vi "Bar Code Reader_v6.vi"() -> ()   [LabVIEW 2016]
uses:
  <vilib>/NXT/Block Support/NXT_OutputPort.ctl
  <vilib>/NXT/Block Support/NXT_InputPort.ctl
  <vilib>/NXT/Dual Mode Library/Sensors/EV3_Color_Color.vi
  <vilib>/NXT/NXTIO Xnodes/NXTIONodeSubVIs/NXTMoveMotors.vi
  <vilib>/NXT/NXTIO Xnodes/NXTIONodeSubVIs/NXTMotorRunDistance.vi
  <vilib>/NXT/Dual Mode Library/Waits/Wait_Num.vi
  <vilib>/NXT/Subs/LVHSConnector.ctl
  <vilib>/NXT/NXTIO Xnodes/AddressXNode/NXTIOAddress.xnode
  <vilib>/NXT/NXTIO Xnodes/NXTIOXNode/NXTIO.xnode
  <vilib>/NXT/LegoClasses/BrickReference/BrickReference.lvclass
panel:
  out "Error Message":string
  out "Total Marbles":dbl
  out "Small/HDPE 4":dbl
  out "Large/Steel 4":dbl
  out "Material 4":string
  out "Small/HDPE 3":dbl
  out "Large/Steel 3":dbl
  out "Material 3":string
  out "Small/HDPE 2":dbl
  out "Large/Steel 2":dbl
  out "Material 2":string
  out "Small/HDPE 1":dbl
  out "Large/Steel 1":dbl
  out "String 3":string
  out "String 2":string
  out "Material 1":string
  out "String":string
  out "Numeric":dbl
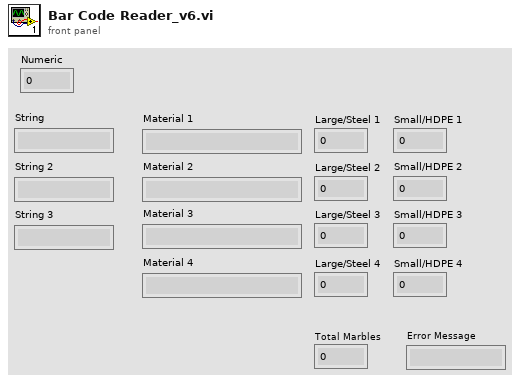
[diagram p1: front panel]
types:
  T1 = typedef "NXT_OutputPort.ctl" = u8
  T2 = typedef "ColorSensorColors.ctl" = enum16{"No Color", "Black", "Blue", "Green", "Yellow", "Red", "White", "Brown"}
  T3 = typedef "LVHSConnector.ctl" = refnum<class "BrickReference.lvclass">
  T4 = typedef "NXT_InputPort.ctl" = u32
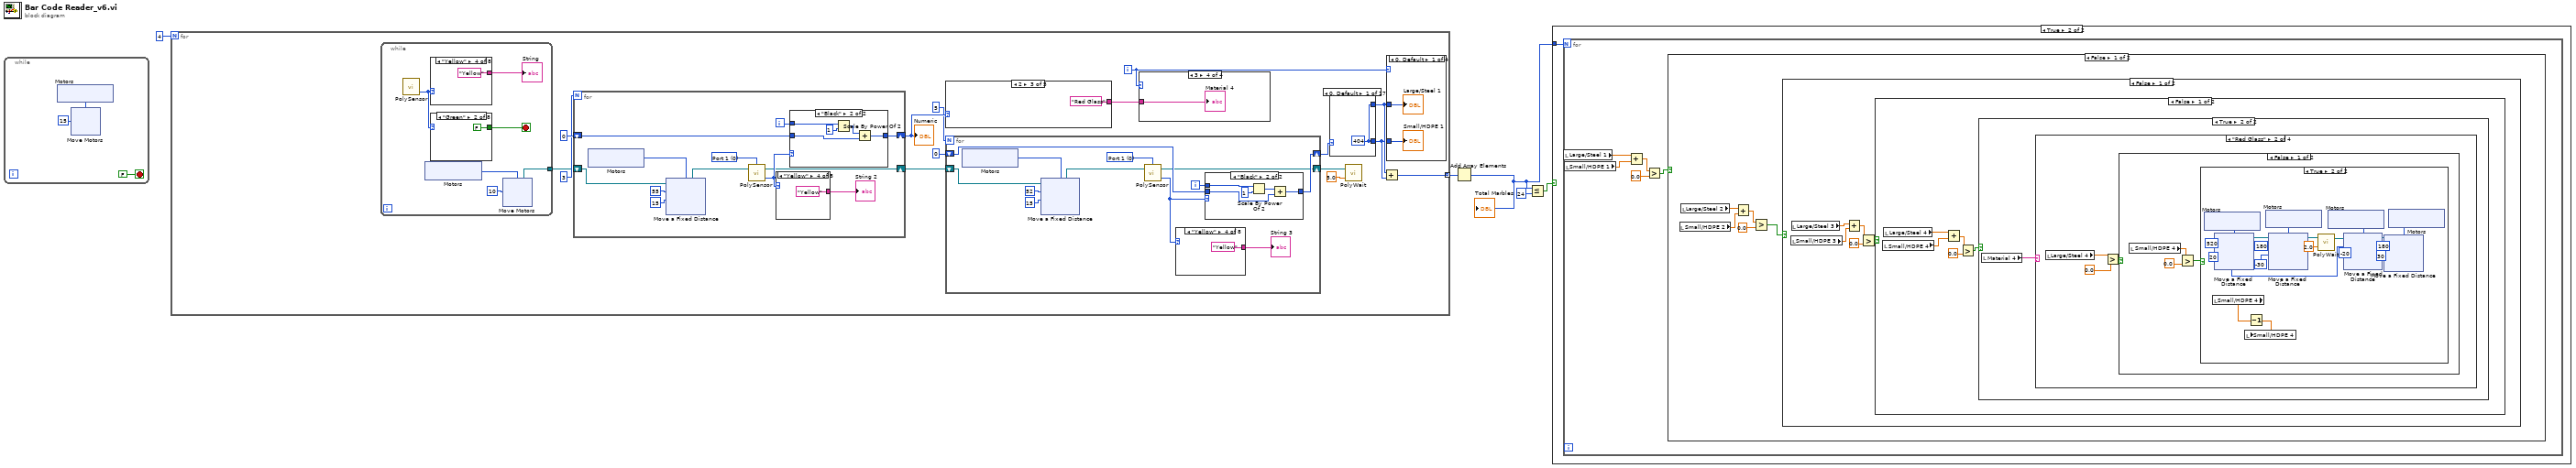
[diagram p0: block diagram]
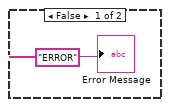
[diagram p2: hidden frame]
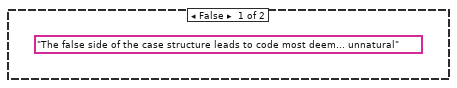
[diagram p3: hidden frame]
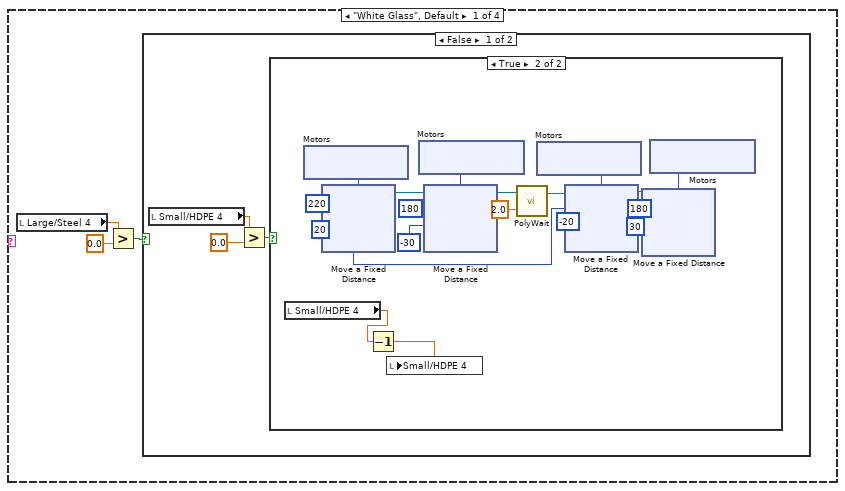
[diagram p4: hidden frame]
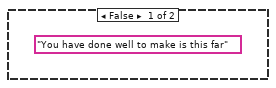
[diagram p5: hidden frame]
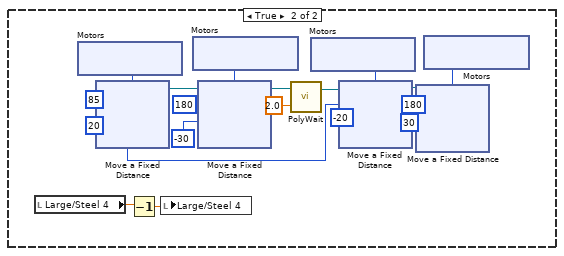
[diagram p6: hidden frame]
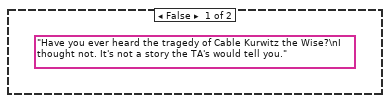
[diagram p7: hidden frame]
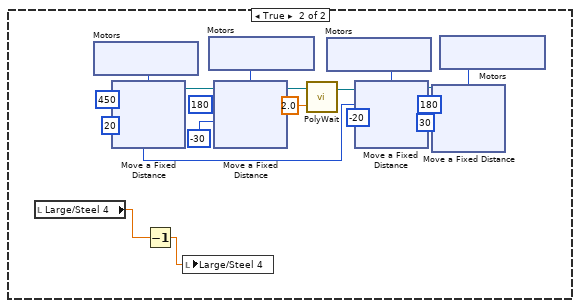
[diagram p8: hidden frame]
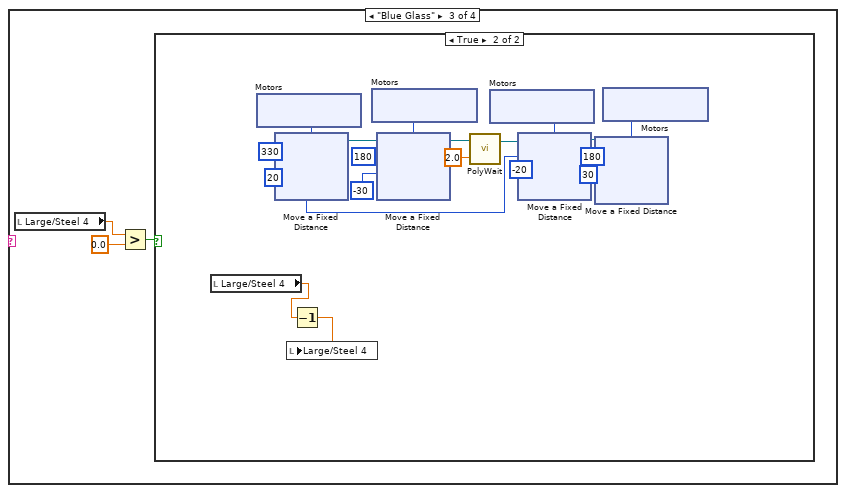
[diagram p9: hidden frame]
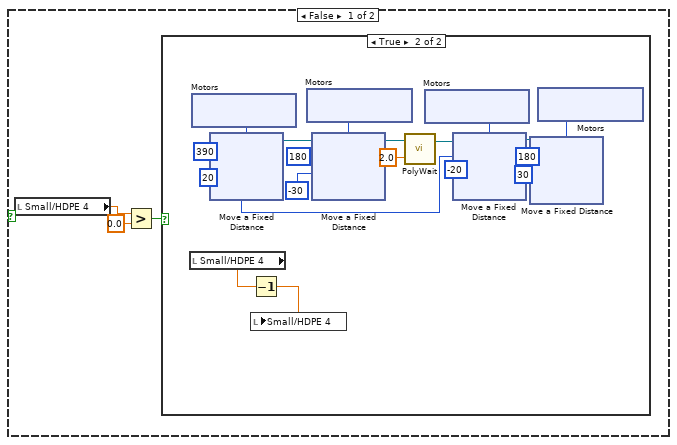
[diagram p10: hidden frame]
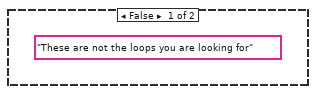
[diagram p11: hidden frame]
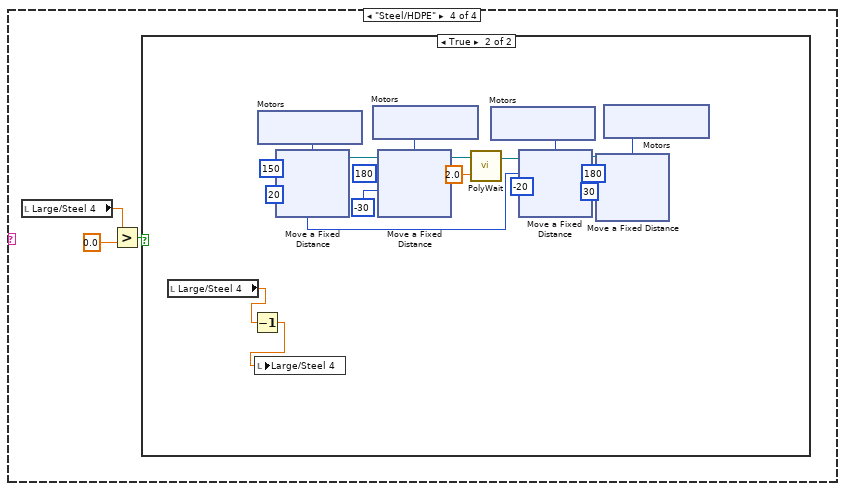
[diagram p12: hidden frame]
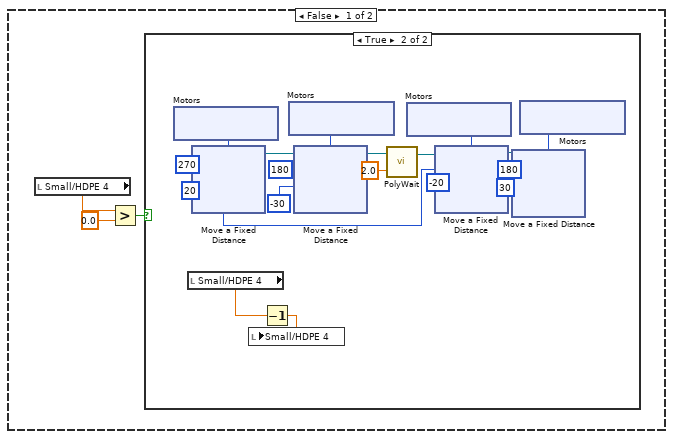
[diagram p13: hidden frame]
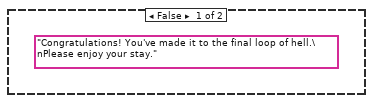
[diagram p14: hidden frame]
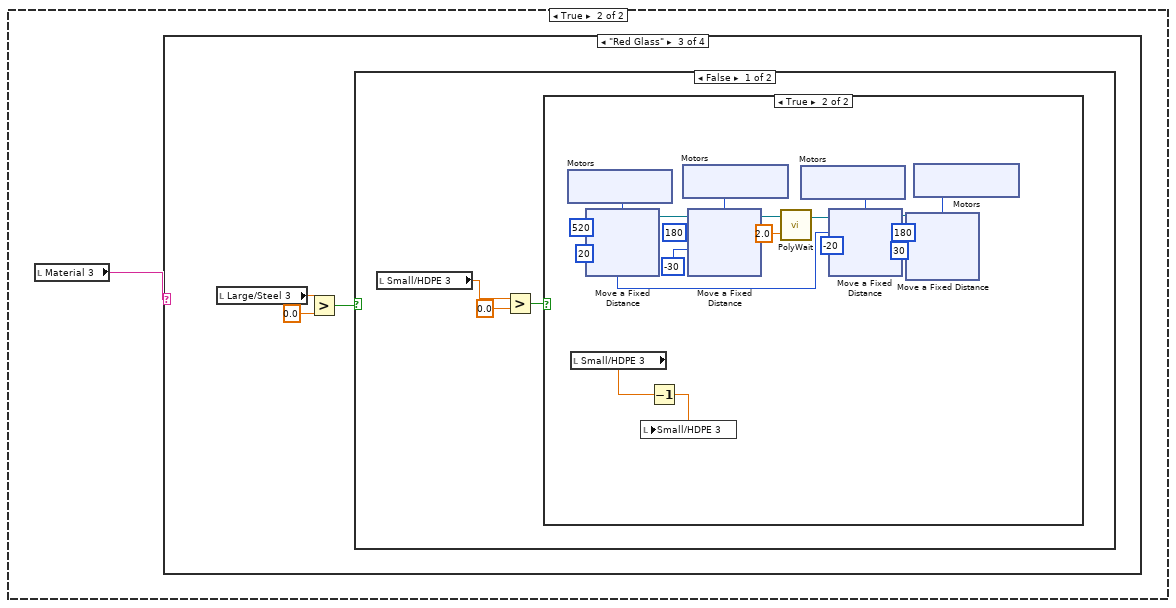
[diagram p15: hidden frame]
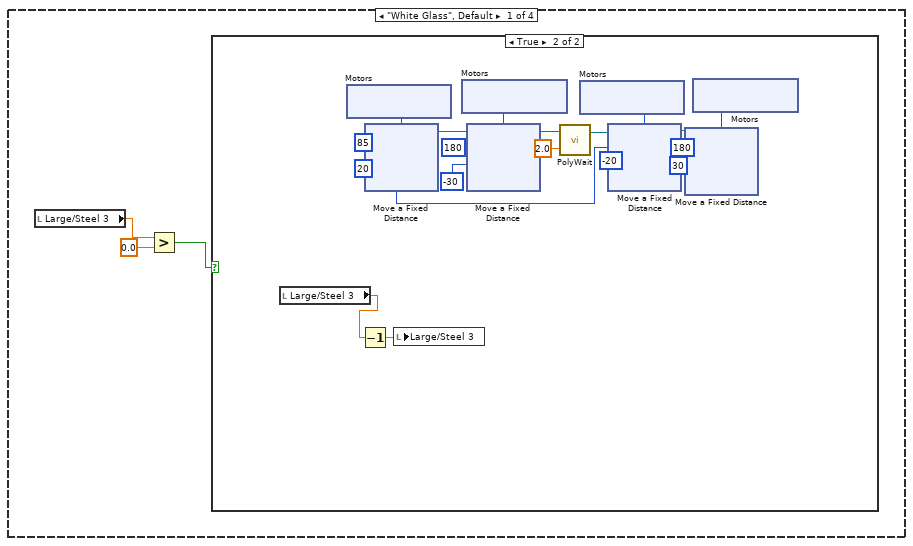
[diagram p16: hidden frame]
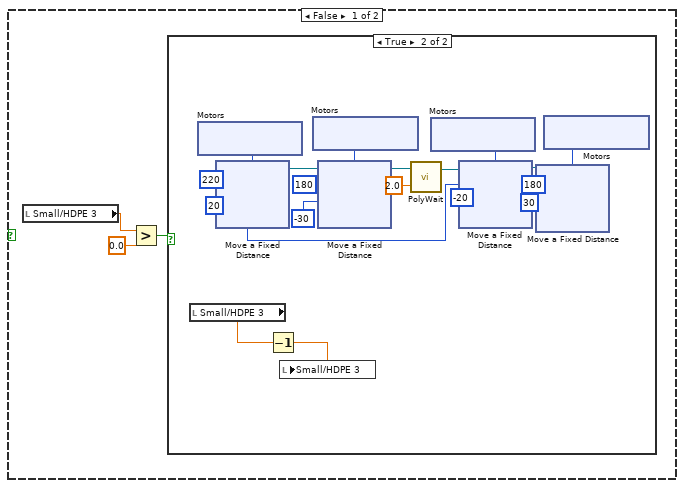
[diagram p17: hidden frame]
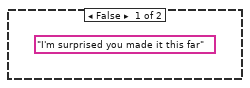
[diagram p18: hidden frame]
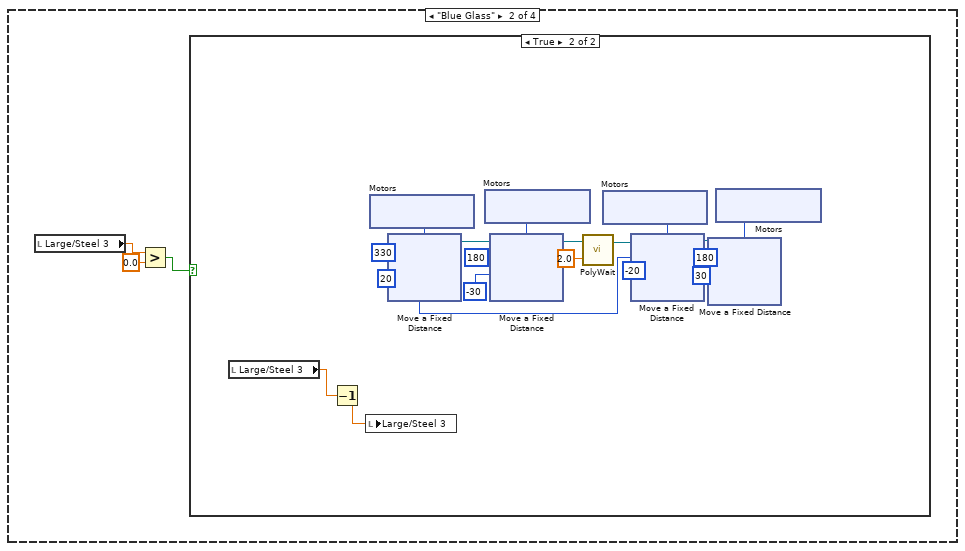
[diagram p19: hidden frame]
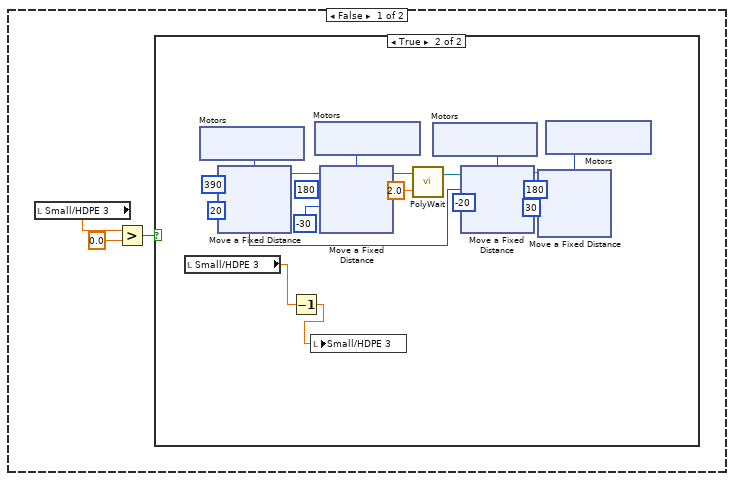
[diagram p20: hidden frame]
diagram:
  n1 = while {
    stop <- FALSE stop-if-true
    n2 = xnode "Motors"() -> ("Motor"=w6:T1)
    n3 = xnode "Move Motors"("Power/Speed 1"=i8 15, "Motors"=w6) -> ()  [unwired: 1 in, 1 out]
  }
  n4 = for {
    N: 4 -> [_]
    tunnel: [w17] -> w4 mode=indexing
    i -> [w22]
    n5 = while {
      tunnel: [w120] -> w29
      stop <- w124 stop-if-true
      n6 = call-poly <vilib>:"PolySensor.vi"() -> ("Detected Color"=w122:T2)  [unwired: 3 in, 1 out]
      n7 = xnode "Motors"() -> ("Motor"=w119:T1)
      n8 = case shown="\"Yellow\"" w122 {
        tunnel: ["No Color" "Blue" "Green" "Yellow" "Red" "White" "Brown" "Black"] -> w123
        frame "No Color", Default {
        }
        frame "Blue" {
        }
        frame "Green" {
        }
        frame "Yellow" {
        }
        frame "Red" {
        }
        frame "White" {
        }
        frame "Brown" {
        }
        frame "Black" {
        }
      }
      "String" <- w123
      n9 = case shown="\"Green\"" w122 {
        tunnel: [FALSE FALSE FALSE FALSE FALSE FALSE FALSE TRUE] -> w124
        frame "No Color", Default {
        }
        frame "Green" {
        }
        frame "Yellow" {
        }
        frame "Red" {
        }
        frame "White" {
        }
        frame "Brown" {
        }
        frame "Blue" {
        }
        frame "Black" {
        }
      }
      n10 = xnode "Move Motors"("Power/Speed 1"=i8 10, "Motors"=w119) -> ("NXT/EV3"=w120:T3)  [unwired: 1 in]
    }
    n11 = for {
      N: 3 -> [_]
      shift-right: [w160] -> w28
      shift-left: 0 -> [w159]
      shift-right: [w155] -> w24
      shift-left: w29 -> [w152]
      i -> [w156]
      w149 = T4 0 items=["Port 1", "Port 2", "Port 3", "Port 4"] ("Port (Port 1)")
      n12 = xnode "Motors"() -> ("Motor"=w150:T1)
      n13 = xnode "Move a Fixed Distance"("Speed 1"=i8 15, "Distance 1"=55, "Motors"=w150, "NXT/EV3"=w152) -> ("NXT/EV3"=w151:T3)
      n14 = call-poly <vilib>:"PolySensor.vi"("NXT/EV3"=w151, "Port (Port 1)"=w149) -> ("Detected Color"=w157:T2, "NXT/EV3"=w155:T3)  [unwired: 1 in]
      n15 = case shown="\"Yellow\"" w157 {
        tunnel: ["No Color" "Blue" "Green" "Yellow" "Red" "White" "Brown" "Black"] -> w158
        frame "No Color", Default {
        }
        frame "Blue" {
        }
        frame "Green" {
        }
        frame "Yellow" {
        }
        frame "Red" {
        }
        frame "White" {
        }
        frame "Brown" {
        }
        frame "Black" {
        }
      }
      "String 2" <- w158
      n16 = case shown="\"Black\"" w157 {
        tunnel: w156 -> [_ w184]
        tunnel: [w180 w182] -> w160
        tunnel: w159 -> [w180 w181]
        frame "White", Default {
        }
        frame "Black" {
          n17 = Scale By Power Of 2(n=w184, x=1) -> (x*2^n=w183:i32)
          n18 = Add(x=w183, y=w181) -> (x+y=w182:i32)
        }
      }
    }
    "Numeric" <- w28
    n19 = case shown="2" w28 {
      tunnel: ["Something has gone wrong" "White Glass" "Red Glass" "Blue Glass" "Steel/HDPE"] -> w27
      frame 0, Default {
      }
      frame 1 {
      }
      frame 2 {
      }
      frame 3 {
      }
      frame 4 {
      }
    }
    n20 = for {
      N: 5 -> [_]
      shift-right: [w88] -> w23
      shift-left: 0 -> [w87]
      shift-right: [w83] -> w21
      shift-left: w24 -> [w80]
      i -> [w84]
      w77 = T4 0 items=["Port 1", "Port 2", "Port 3", "Port 4"] ("Port (Port 1)")
      n21 = xnode "Motors"() -> ("Motor"=w78:T1)
      n22 = xnode "Move a Fixed Distance"("Speed 1"=i8 15, "Distance 1"=52, "Motors"=w78, "NXT/EV3"=w80) -> ("NXT/EV3"=w79:T3)
      n23 = call-poly <vilib>:"PolySensor.vi"("NXT/EV3"=w79, "Port (Port 1)"=w77) -> ("Detected Color"=w85:T2, "NXT/EV3"=w83:T3)  [unwired: 1 in]
      n24 = case shown="\"Yellow\"" w85 {
        tunnel: ["No Color" "Blue" "Green" "Yellow" "Red" "White" "Brown" "Black"] -> w86
        frame "No Color", Default {
        }
        frame "Blue" {
        }
        frame "Green" {
        }
        frame "Yellow" {
        }
        frame "Red" {
        }
        frame "White" {
        }
        frame "Brown" {
        }
        frame "Black" {
        }
      }
      "String 3" <- w86
      n25 = case shown="\"Black\"" w85 {
        tunnel: w84 -> [_ w112]
        tunnel: [w108 w110] -> w88
        tunnel: w87 -> [w108 w109]
        frame "White", Default {
        }
        frame "Black" {
          n26 = Scale By Power Of 2(n=w112, x=1) -> (x*2^n=w111:i32)
          n27 = Add(x=w111, y=w109) -> (x+y=w110:i32)
        }
      }
    }
    n28 = case shown="3" w22 {
      tunnel: w27 -> [w40 w41 w42 w43]
      frame 0, Default {
        "Material 1" <- w40
      }
      frame 1 {
        "Material 2" <- w41
      }
      frame 2 {
        "Material 3" <- w42
      }
      frame 3 {
        "Material 4" <- w43
      }
    }
    n29 = case shown="0, Default" w23 {
      tunnel: [w44 0 1 2 3 0 1 2 3 0 1 2 3 0 1 2 3] -> w19
      tunnel: [w44 0 0 0 0 1 1 1 1 2 2 2 2 3 3 3 3] -> w18
      frame 0, Default {
        w44 = 404
      }
      frame 1 {
      }
      frame 2 {
      }
      frame 3 {
      }
      frame 4 {
      }
      frame 5 {
      }
      frame 6 {
      }
      frame 7 {
      }
      frame 8 {
      }
      frame 9 {
      }
      frame 10 {
      }
      frame 11 {
      }
      frame 12 {
      }
      frame 13 {
      }
      frame 14 {
      }
      frame 15 {
      }
      frame 16 {
      }
    }
    n30 = call-poly <vilib>:"PolyWait.vi"("Time (1 sec)"=sgl 5.0, "NXT/EV3"=w21) -> ()  [unwired: 2 in, 1 out]
    n31 = Add(x=w19, y=w18) -> (x+y=w17:i32)
    n32 = case shown="0, Default" w22 {
      tunnel: w19 -> [w33 w34 w36 w38]
      tunnel: w18 -> [w32 w35 w37 w39]
      frame 0, Default {
        "Small/HDPE 1" <- w32
        "Large/Steel 1" <- w33
      }
      frame 1 {
        "Large/Steel 2" <- w34
        "Small/HDPE 2" <- w35
      }
      frame 2 {
        "Large/Steel 3" <- w36
        "Small/HDPE 3" <- w37
      }
      frame 3 {
        "Large/Steel 4" <- w38
        "Small/HDPE 4" <- w39
      }
    }
  }
  n33 = Add Array Elements(numeric array=w4) -> (sum=w3:i32)
  "Total Marbles" <- w3
  n34 = Less Or Equal?(x=w3, y=24) -> (x <= y?=w1:bool)
  n35 = case shown="True" w1 {
    tunnel: w3 -> [_ w187]
    frame False {
      "Error Message" <- "ERROR"
    }
    frame True {
      n36 = for {
        N: w187 -> [_]
        n37 = local read "Large/Steel 1"() -> (w192:dbl)
        n38 = local read "Small/HDPE 1"() -> (w191:dbl)
        n39 = Add(x=w192, y=w191) -> (x+y=w190:dbl)
        n40 = Greater?(x=w190, y=0.0) -> (0:w188:bool)
        n41 = case shown="False" w188 {
          frame False {
            n42 = local read "Small/HDPE 2"() -> (w195:dbl)
            n43 = local read "Large/Steel 2"() -> (w194:dbl)
            n44 = Add(x=w194, y=w195) -> (x+y=w197:dbl)
            n45 = Greater?(x=w197, y=0.0) -> (0:w193:bool)
            n46 = case shown="False" w193 {
              frame False {
                n47 = local read "Small/HDPE 3"() -> (w199:dbl)
                n48 = local read "Large/Steel 3"() -> (w200:dbl)
                n49 = Add(x=w200, y=w199) -> (x+y=w202:dbl)
                n50 = Greater?(x=w202, y=0.0) -> (0:w198:bool)
                n51 = case shown="False" w198 {
                  frame False {
                    n52 = local read "Small/HDPE 4"() -> (w204:dbl)
                    n53 = local read "Large/Steel 4"() -> (w205:dbl)
                    n54 = Add(x=w205, y=w204) -> (x+y=w207:dbl)
                    n55 = Greater?(x=w207, y=0.0) -> (0:w203:bool)
                    n56 = case shown="True" w203 {
                      frame False {
                        (unwired) "The false side of the case structure leads to code most deem... unnatural"
                      }
                      frame True {
                        n57 = local read "Material 4"() -> (w208:string)
                        n58 = case shown="\"Red Glass\"" w208 {
                          frame "White Glass", Default {
                            n59 = local read "Large/Steel 4"() -> (w210:dbl)
                            n60 = Greater?(x=w210, y=0.0) -> (0:w211:bool)
                            n61 = case shown="False" w211 {
                              frame False {
                                n62 = local read "Small/HDPE 4"() -> (w213:dbl)
                                n63 = Greater?(x=w213, y=0.0) -> (0:w214:bool)
                                n64 = case shown="True" w214 {
                                frame False {
                                (unwired) "You have done well to make is this far"
                                }
                                frame True {
                                w221 = 220 ("Distance 1")
                                n65 = local read "Small/HDPE 4"() -> (w232:dbl)
                                n66 = xnode "Motors"() -> ("Motor"=w222:T1)
                                n67 = xnode "Move a Fixed Distance"("Speed 1"=i8 20, "Distance 1"=w221, "Motors"=w222) -> ("NXT/EV3"=w216:T3)  [unwired: 1 in]
                                n68 = Decrement(x=w232) -> (x-1=w231:dbl)
                                n69 = local write "Small/HDPE 4"(w231) -> ()
                                n70 = xnode "Motors"() -> ("Motor"=w224:T1)
                                n71 = xnode "Move a Fixed Distance"("Speed 1"=i8 -30, "Distance 1"=180, "Motors"=w224, "NXT/EV3"=w216) -> ("NXT/EV3"=w215:T3)
                                n72 = call-poly <vilib>:"PolyWait.vi"("Time (1 sec)"=sgl 2.0, "NXT/EV3"=w215) -> ("NXT/EV3"=w217:T3)  [unwired: 2 in]
                                n73 = xnode "Motors"() -> ("Motor"=w219:T1)
                                n74 = xnode "Move a Fixed Distance"("Speed 1"=i8 -20, "Distance 1"=w221, "Motors"=w219, "NXT/EV3"=w217) -> ("NXT/EV3"=w220:T3)
                                n75 = xnode "Motors"() -> ("Motor"=w227:T1)
                                n76 = xnode "Move a Fixed Distance"("Speed 1"=i8 30, "Distance 1"=180, "Motors"=w227, "NXT/EV3"=w220) -> ()  [unwired: 1 out]
                                }
                                }
                              }
                              frame True {
                                w283 = 85 ("Distance 1")
                                n77 = local read "Large/Steel 4"() -> (w294:dbl)
                                n78 = xnode "Motors"() -> ("Motor"=w284:T1)
                                n79 = xnode "Move a Fixed Distance"("Speed 1"=i8 20, "Distance 1"=w283, "Motors"=w284) -> ("NXT/EV3"=w278:T3)  [unwired: 1 in]
                                n80 = Decrement(x=w294) -> (x-1=w293:dbl)
                                n81 = local write "Large/Steel 4"(w293) -> ()
                                n82 = xnode "Motors"() -> ("Motor"=w286:T1)
                                n83 = xnode "Move a Fixed Distance"("Speed 1"=i8 -30, "Distance 1"=180, "Motors"=w286, "NXT/EV3"=w278) -> ("NXT/EV3"=w277:T3)
                                n84 = call-poly <vilib>:"PolyWait.vi"("Time (1 sec)"=sgl 2.0, "NXT/EV3"=w277) -> ("NXT/EV3"=w279:T3)  [unwired: 2 in]
                                n85 = xnode "Motors"() -> ("Motor"=w281:T1)
                                n86 = xnode "Move a Fixed Distance"("Speed 1"=i8 -20, "Distance 1"=w283, "Motors"=w281, "NXT/EV3"=w279) -> ("NXT/EV3"=w282:T3)
                                n87 = xnode "Motors"() -> ("Motor"=w289:T1)
                                n88 = xnode "Move a Fixed Distance"("Speed 1"=i8 30, "Distance 1"=180, "Motors"=w289, "NXT/EV3"=w282) -> ()  [unwired: 1 out]
                              }
                            }
                          }
                          frame "Red Glass" {
                            n89 = local read "Large/Steel 4"() -> (w340:dbl)
                            n90 = Greater?(x=w340, y=0.0) -> (0:w341:bool)
                            n91 = case shown="False" w341 {
                              frame False {
                                n92 = local read "Small/HDPE 4"() -> (w342:dbl)
                                n93 = Greater?(x=w342, y=0.0) -> (0:w344:bool)
                                n94 = case shown="True" w344 {
                                frame False {
                                (unwired) "Have you ever heard the tragedy of Cable Kurwitz the Wise?\nI thought not. It's not a story the TA's would tell you."
                                }
                                frame True {
                                w351 = 520 ("Distance 1")
                                n95 = xnode "Motors"() -> ("Motor"=w352:T1)
                                n96 = local read "Small/HDPE 4"() -> (w362:dbl)
                                n97 = xnode "Move a Fixed Distance"("Speed 1"=i8 20, "Distance 1"=w351, "Motors"=w352) -> ("NXT/EV3"=w346:T3)  [unwired: 1 in]
                                n98 = Decrement(x=w362) -> (x-1=w361:dbl)
                                n99 = local write "Small/HDPE 4"(w361) -> ()
                                n100 = xnode "Motors"() -> ("Motor"=w354:T1)
                                n101 = xnode "Move a Fixed Distance"("Speed 1"=i8 -30, "Distance 1"=180, "Motors"=w354, "NXT/EV3"=w346) -> ("NXT/EV3"=w345:T3)
                                n102 = call-poly <vilib>:"PolyWait.vi"("Time (1 sec)"=sgl 2.0, "NXT/EV3"=w345) -> ("NXT/EV3"=w347:T3)  [unwired: 2 in]
                                n103 = xnode "Motors"() -> ("Motor"=w349:T1)
                                n104 = xnode "Move a Fixed Distance"("Speed 1"=i8 -20, "Distance 1"=w351, "Motors"=w349, "NXT/EV3"=w347) -> ("NXT/EV3"=w350:T3)
                                n105 = xnode "Motors"() -> ("Motor"=w357:T1)
                                n106 = xnode "Move a Fixed Distance"("Speed 1"=i8 30, "Distance 1"=180, "Motors"=w357, "NXT/EV3"=w350) -> ()  [unwired: 1 out]
                                }
                                }
                              }
                              frame True {
                                w413 = 450 ("Distance 1")
                                n107 = local read "Large/Steel 4"() -> (w424:dbl)
                                n108 = xnode "Motors"() -> ("Motor"=w414:T1)
                                n109 = xnode "Move a Fixed Distance"("Speed 1"=i8 20, "Distance 1"=w413, "Motors"=w414) -> ("NXT/EV3"=w408:T3)  [unwired: 1 in]
                                n110 = Decrement(x=w424) -> (x-1=w423:dbl)
                                n111 = local write "Large/Steel 4"(w423) -> ()
                                n112 = xnode "Motors"() -> ("Motor"=w416:T1)
                                n113 = xnode "Move a Fixed Distance"("Speed 1"=i8 -30, "Distance 1"=180, "Motors"=w416, "NXT/EV3"=w408) -> ("NXT/EV3"=w407:T3)
                                n114 = call-poly <vilib>:"PolyWait.vi"("Time (1 sec)"=sgl 2.0, "NXT/EV3"=w407) -> ("NXT/EV3"=w409:T3)  [unwired: 2 in]
                                n115 = xnode "Motors"() -> ("Motor"=w411:T1)
                                n116 = xnode "Move a Fixed Distance"("Speed 1"=i8 -20, "Distance 1"=w413, "Motors"=w411, "NXT/EV3"=w409) -> ("NXT/EV3"=w412:T3)
                                n117 = xnode "Motors"() -> ("Motor"=w419:T1)
                                n118 = xnode "Move a Fixed Distance"("Speed 1"=i8 30, "Distance 1"=180, "Motors"=w419, "NXT/EV3"=w412) -> ()  [unwired: 1 out]
                              }
                            }
                          }
                          frame "Blue Glass" {
                            n119 = local read "Large/Steel 4"() -> (w471:dbl)
                            n120 = Greater?(x=w471, y=0.0) -> (0:w470:bool)
                            n121 = case shown="True" w470 {
                              frame False {
                                n122 = local read "Small/HDPE 4"() -> (w473:dbl)
                                n123 = Greater?(x=w473, y=0.0) -> (0:w474:bool)
                                n124 = case shown="True" w474 {
                                frame False {
                                (unwired) "These are not the loops you are looking for"
                                }
                                frame True {
                                w481 = 390 ("Distance 1")
                                n125 = local read "Small/HDPE 4"() -> (w492:dbl)
                                n126 = xnode "Motors"() -> ("Motor"=w482:T1)
                                n127 = xnode "Move a Fixed Distance"("Speed 1"=i8 20, "Distance 1"=w481, "Motors"=w482) -> ("NXT/EV3"=w476:T3)  [unwired: 1 in]
                                n128 = Decrement(x=w492) -> (x-1=w491:dbl)
                                n129 = local write "Small/HDPE 4"(w491) -> ()
                                n130 = xnode "Motors"() -> ("Motor"=w484:T1)
                                n131 = xnode "Move a Fixed Distance"("Speed 1"=i8 -30, "Distance 1"=180, "Motors"=w484, "NXT/EV3"=w476) -> ("NXT/EV3"=w475:T3)
                                n132 = call-poly <vilib>:"PolyWait.vi"("Time (1 sec)"=sgl 2.0, "NXT/EV3"=w475) -> ("NXT/EV3"=w477:T3)  [unwired: 2 in]
                                n133 = xnode "Motors"() -> ("Motor"=w479:T1)
                                n134 = xnode "Move a Fixed Distance"("Speed 1"=i8 -20, "Distance 1"=w481, "Motors"=w479, "NXT/EV3"=w477) -> ("NXT/EV3"=w480:T3)
                                n135 = xnode "Motors"() -> ("Motor"=w487:T1)
                                n136 = xnode "Move a Fixed Distance"("Speed 1"=i8 30, "Distance 1"=180, "Motors"=w487, "NXT/EV3"=w480) -> ()  [unwired: 1 out]
                                }
                                }
                              }
                              frame True {
                                w543 = 330 ("Distance 1")
                                n137 = local read "Large/Steel 4"() -> (w554:dbl)
                                n138 = xnode "Motors"() -> ("Motor"=w544:T1)
                                n139 = xnode "Move a Fixed Distance"("Speed 1"=i8 20, "Distance 1"=w543, "Motors"=w544) -> ("NXT/EV3"=w538:T3)  [unwired: 1 in]
                                n140 = Decrement(x=w554) -> (x-1=w553:dbl)
                                n141 = local write "Large/Steel 4"(w553) -> ()
                                n142 = xnode "Motors"() -> ("Motor"=w546:T1)
                                n143 = xnode "Move a Fixed Distance"("Speed 1"=i8 -30, "Distance 1"=180, "Motors"=w546, "NXT/EV3"=w538) -> ("NXT/EV3"=w537:T3)
                                n144 = call-poly <vilib>:"PolyWait.vi"("Time (1 sec)"=sgl 2.0, "NXT/EV3"=w537) -> ("NXT/EV3"=w539:T3)  [unwired: 2 in]
                                n145 = xnode "Motors"() -> ("Motor"=w541:T1)
                                n146 = xnode "Move a Fixed Distance"("Speed 1"=i8 -20, "Distance 1"=w543, "Motors"=w541, "NXT/EV3"=w539) -> ("NXT/EV3"=w542:T3)
                                n147 = xnode "Motors"() -> ("Motor"=w549:T1)
                                n148 = xnode "Move a Fixed Distance"("Speed 1"=i8 30, "Distance 1"=180, "Motors"=w549, "NXT/EV3"=w542) -> ()  [unwired: 1 out]
                              }
                            }
                          }
                          frame "Steel/HDPE" {
                            n149 = local read "Large/Steel 4"() -> (w600:dbl)
                            n150 = Greater?(x=w600, y=0.0) -> (0:w601:bool)
                            n151 = case shown="True" w601 {
                              frame False {
                                n152 = local read "Small/HDPE 4"() -> (w603:dbl)
                                n153 = Greater?(x=w603, y=0.0) -> (0:w604:bool)
                                n154 = case shown="True" w604 {
                                frame False {
                                (unwired) "Congratulations! You've made it to the final loop of hell.\nPlease enjoy your stay."
                                }
                                frame True {
                                w611 = 270 ("Distance 1")
                                n155 = xnode "Motors"() -> ("Motor"=w612:T1)
                                n156 = local read "Small/HDPE 4"() -> (w622:dbl)
                                n157 = xnode "Move a Fixed Distance"("Speed 1"=i8 20, "Distance 1"=w611, "Motors"=w612) -> ("NXT/EV3"=w606:T3)  [unwired: 1 in]
                                n158 = Decrement(x=w622) -> (x-1=w621:dbl)
                                n159 = local write "Small/HDPE 4"(w621) -> ()
                                n160 = xnode "Motors"() -> ("Motor"=w614:T1)
                                n161 = xnode "Move a Fixed Distance"("Speed 1"=i8 -30, "Distance 1"=180, "Motors"=w614, "NXT/EV3"=w606) -> ("NXT/EV3"=w605:T3)
                                n162 = call-poly <vilib>:"PolyWait.vi"("Time (1 sec)"=sgl 2.0, "NXT/EV3"=w605) -> ("NXT/EV3"=w607:T3)  [unwired: 2 in]
                                n163 = xnode "Motors"() -> ("Motor"=w609:T1)
                                n164 = xnode "Move a Fixed Distance"("Speed 1"=i8 -20, "Distance 1"=w611, "Motors"=w609, "NXT/EV3"=w607) -> ("NXT/EV3"=w610:T3)
                                n165 = xnode "Motors"() -> ("Motor"=w617:T1)
                                n166 = xnode "Move a Fixed Distance"("Speed 1"=i8 30, "Distance 1"=180, "Motors"=w617, "NXT/EV3"=w610) -> ()  [unwired: 1 out]
                                }
                                }
                              }
                              frame True {
                                w673 = 150 ("Distance 1")
                                n167 = local read "Large/Steel 4"() -> (w684:dbl)
                                n168 = Decrement(x=w684) -> (x-1=w683:dbl)
                                n169 = local write "Large/Steel 4"(w683) -> ()
                                n170 = xnode "Motors"() -> ("Motor"=w674:T1)
                                n171 = xnode "Move a Fixed Distance"("Speed 1"=i8 20, "Distance 1"=w673, "Motors"=w674) -> ("NXT/EV3"=w668:T3)  [unwired: 1 in]
                                n172 = xnode "Motors"() -> ("Motor"=w676:T1)
                                n173 = xnode "Move a Fixed Distance"("Speed 1"=i8 -30, "Distance 1"=180, "Motors"=w676, "NXT/EV3"=w668) -> ("NXT/EV3"=w667:T3)
                                n174 = call-poly <vilib>:"PolyWait.vi"("Time (1 sec)"=sgl 2.0, "NXT/EV3"=w667) -> ("NXT/EV3"=w669:T3)  [unwired: 2 in]
                                n175 = xnode "Motors"() -> ("Motor"=w671:T1)
                                n176 = xnode "Move a Fixed Distance"("Speed 1"=i8 -20, "Distance 1"=w673, "Motors"=w671, "NXT/EV3"=w669) -> ("NXT/EV3"=w672:T3)
                                n177 = xnode "Motors"() -> ("Motor"=w679:T1)
                                n178 = xnode "Move a Fixed Distance"("Speed 1"=i8 30, "Distance 1"=180, "Motors"=w679, "NXT/EV3"=w672) -> ()  [unwired: 1 out]
                              }
                            }
                          }
                        }
                      }
                    }
                  }
                  frame True {
                    n179 = local read "Material 3"() -> (w729:string)
                    n180 = case shown="\"Red Glass\"" w729 {
                      frame "White Glass", Default {
                        n181 = local read "Large/Steel 3"() -> (w732:dbl)
                        n182 = Greater?(x=w732, y=0.0) -> (0:w730:bool)
                        n183 = case shown="True" w730 {
                          frame False {
                            n184 = local read "Small/HDPE 3"() -> (w734:dbl)
                            n185 = Greater?(x=w734, y=0.0) -> (0:w735:bool)
                            n186 = case shown="True" w735 {
                              frame False {
                                (unwired) "I'm surprised you made it this far"
                              }
                              frame True {
                                w742 = 220 ("Distance 1")
                                n187 = local read "Small/HDPE 3"() -> (w753:dbl)
                                n188 = xnode "Motors"() -> ("Motor"=w743:T1)
                                n189 = xnode "Move a Fixed Distance"("Speed 1"=i8 20, "Distance 1"=w742, "Motors"=w743) -> ("NXT/EV3"=w737:T3)  [unwired: 1 in]
                                n190 = Decrement(x=w753) -> (x-1=w752:dbl)
                                n191 = local write "Small/HDPE 3"(w752) -> ()
                                n192 = xnode "Motors"() -> ("Motor"=w745:T1)
                                n193 = xnode "Move a Fixed Distance"("Speed 1"=i8 -30, "Distance 1"=180, "Motors"=w745, "NXT/EV3"=w737) -> ("NXT/EV3"=w736:T3)
                                n194 = call-poly <vilib>:"PolyWait.vi"("Time (1 sec)"=sgl 2.0, "NXT/EV3"=w736) -> ("NXT/EV3"=w738:T3)  [unwired: 2 in]
                                n195 = xnode "Motors"() -> ("Motor"=w740:T1)
                                n196 = xnode "Move a Fixed Distance"("Speed 1"=i8 -20, "Distance 1"=w742, "Motors"=w740, "NXT/EV3"=w738) -> ("NXT/EV3"=w741:T3)
                                n197 = xnode "Motors"() -> ("Motor"=w748:T1)
                                n198 = xnode "Move a Fixed Distance"("Speed 1"=i8 30, "Distance 1"=180, "Motors"=w748, "NXT/EV3"=w741) -> ()  [unwired: 1 out]
                              }
                            }
                          }
                          frame True {
                            w804 = 85 ("Distance 1")
                            n199 = local read "Large/Steel 3"() -> (w815:dbl)
                            n200 = xnode "Motors"() -> ("Motor"=w805:T1)
                            n201 = Decrement(x=w815) -> (x-1=w814:dbl)
                            n202 = xnode "Move a Fixed Distance"("Speed 1"=i8 20, "Distance 1"=w804, "Motors"=w805) -> ("NXT/EV3"=w799:T3)  [unwired: 1 in]
                            n203 = local write "Large/Steel 3"(w814) -> ()
                            n204 = xnode "Motors"() -> ("Motor"=w807:T1)
                            n205 = xnode "Move a Fixed Distance"("Speed 1"=i8 -30, "Distance 1"=180, "Motors"=w807, "NXT/EV3"=w799) -> ("NXT/EV3"=w798:T3)
                            n206 = call-poly <vilib>:"PolyWait.vi"("Time (1 sec)"=sgl 2.0, "NXT/EV3"=w798) -> ("NXT/EV3"=w800:T3)  [unwired: 2 in]
                            n207 = xnode "Motors"() -> ("Motor"=w802:T1)
                            n208 = xnode "Move a Fixed Distance"("Speed 1"=i8 -20, "Distance 1"=w804, "Motors"=w802, "NXT/EV3"=w800) -> ("NXT/EV3"=w803:T3)
                            n209 = xnode "Motors"() -> ("Motor"=w810:T1)
                            n210 = xnode "Move a Fixed Distance"("Speed 1"=i8 30, "Distance 1"=180, "Motors"=w810, "NXT/EV3"=w803) -> ()  [unwired: 1 out]
                          }
                        }
                      }
                      frame "Blue Glass" {
                        n211 = local read "Large/Steel 3"() -> (w862:dbl)
                        n212 = Greater?(x=w862, y=0.0) -> (0:w860:bool)
                        n213 = case shown="True" w860 {
                          frame False {
                            n214 = local read "Small/HDPE 3"() -> (w865:dbl)
                            n215 = Greater?(x=w865, y=0.0) -> (0:w863:bool)
                            n216 = case shown="True" w863 {
                              frame False {
                                (unwired) "Welcome to the dark side of the case structure"
                              }
                              frame True {
                                w872 = 390 ("Distance 1")
                                n217 = local read "Small/HDPE 3"() -> (w883:dbl)
                                n218 = xnode "Motors"() -> ("Motor"=w873:T1)
                                n219 = xnode "Move a Fixed Distance"("Speed 1"=i8 20, "Distance 1"=w872, "Motors"=w873) -> ("NXT/EV3"=w867:T3)  [unwired: 1 in]
                                n220 = Decrement(x=w883) -> (x-1=w882:dbl)
                                n221 = local write "Small/HDPE 3"(w882) -> ()
                                n222 = xnode "Motors"() -> ("Motor"=w875:T1)
                                n223 = xnode "Move a Fixed Distance"("Speed 1"=i8 -30, "Distance 1"=180, "Motors"=w875, "NXT/EV3"=w867) -> ("NXT/EV3"=w866:T3)
                                n224 = call-poly <vilib>:"PolyWait.vi"("Time (1 sec)"=sgl 2.0, "NXT/EV3"=w866) -> ("NXT/EV3"=w868:T3)  [unwired: 2 in]
                                n225 = xnode "Motors"() -> ("Motor"=w870:T1)
                                n226 = xnode "Move a Fixed Distance"("Speed 1"=i8 -20, "Distance 1"=w872, "Motors"=w870, "NXT/EV3"=w868) -> ("NXT/EV3"=w871:T3)
                                n227 = xnode "Motors"() -> ("Motor"=w878:T1)
                                n228 = xnode "Move a Fixed Distance"("Speed 1"=i8 30, "Distance 1"=180, "Motors"=w878, "NXT/EV3"=w871) -> ()  [unwired: 1 out]
                              }
                            }
                          }
                          frame True {
                            w934 = 330 ("Distance 1")
                            n229 = local read "Large/Steel 3"() -> (w945:dbl)
                            n230 = Decrement(x=w945) -> (x-1=w944:dbl)
                            n231 = local write "Large/Steel 3"(w944) -> ()
                            n232 = xnode "Motors"() -> ("Motor"=w935:T1)
                            n233 = xnode "Move a Fixed Distance"("Speed 1"=i8 20, "Distance 1"=w934, "Motors"=w935) -> ("NXT/EV3"=w929:T3)  [unwired: 1 in]
                            n234 = xnode "Motors"() -> ("Motor"=w937:T1)
                            n235 = xnode "Move a Fixed Distance"("Speed 1"=i8 -30, "Distance 1"=180, "Motors"=w937, "NXT/EV3"=w929) -> ("NXT/EV3"=w928:T3)
                            n236 = call-poly <vilib>:"PolyWait.vi"("Time (1 sec)"=sgl 2.0, "NXT/EV3"=w928) -> ("NXT/EV3"=w930:T3)  [unwired: 2 in]
                            n237 = xnode "Motors"() -> ("Motor"=w932:T1)
                            n238 = xnode "Move a Fixed Distance"("Speed 1"=i8 -20, "Distance 1"=w934, "Motors"=w932, "NXT/EV3"=w930) -> ("NXT/EV3"=w933:T3)
                            n239 = xnode "Motors"() -> ("Motor"=w940:T1)
                            n240 = xnode "Move a Fixed Distance"("Speed 1"=i8 30, "Distance 1"=180, "Motors"=w940, "NXT/EV3"=w933) -> ()  [unwired: 1 out]
                          }
                        }
                      }
                      frame "Red Glass" {
                        n241 = local read "Large/Steel 3"() -> (w991:dbl)
                        n242 = Greater?(x=w991, y=0.0) -> (0:w992:bool)
                        n243 = case shown="False" w992 {
                          frame False {
                            n244 = local read "Small/HDPE 3"() -> (w994:dbl)
                            n245 = Greater?(x=w994, y=0.0) -> (0:w995:bool)
                            n246 = case shown="True" w995 {
                              frame False {
                                (unwired) "Two to the one to the one to the three"
                              }
                              frame True {
                                w1002 = 520 ("Distance 1")
                                n247 = xnode "Motors"() -> ("Motor"=w1003:T1)
                                n248 = local read "Small/HDPE 3"() -> (w1013:dbl)
                                n249 = xnode "Move a Fixed Distance"("Speed 1"=i8 20, "Distance 1"=w1002, "Motors"=w1003) -> ("NXT/EV3"=w997:T3)  [unwired: 1 in]
                                n250 = Decrement(x=w1013) -> (x-1=w1012:dbl)
                                n251 = local write "Small/HDPE 3"(w1012) -> ()
                                n252 = xnode "Motors"() -> ("Motor"=w1005:T1)
                                n253 = xnode "Move a Fixed Distance"("Speed 1"=i8 -30, "Distance 1"=180, "Motors"=w1005, "NXT/EV3"=w997) -> ("NXT/EV3"=w996:T3)
                                n254 = call-poly <vilib>:"PolyWait.vi"("Time (1 sec)"=sgl 2.0, "NXT/EV3"=w996) -> ("NXT/EV3"=w998:T3)  [unwired: 2 in]
                                n255 = xnode "Motors"() -> ("Motor"=w1000:T1)
                                n256 = xnode "Move a Fixed Distance"("Speed 1"=i8 -20, "Distance 1"=w1002, "Motors"=w1000, "NXT/EV3"=w998) -> ("NXT/EV3"=w1001:T3)
                                n257 = xnode "Motors"() -> ("Motor"=w1008:T1)
                                n258 = xnode "Move a Fixed Distance"("Speed 1"=i8 30, "Distance 1"=180, "Motors"=w1008, "NXT/EV3"=w1001) -> ()  [unwired: 1 out]
                              }
                            }
                          }
                          frame True {
                            w1064 = 450 ("Distance 1")
                            n259 = local read "Large/Steel 3"() -> (w1075:dbl)
                            n260 = Decrement(x=w1075) -> (x-1=w1074:dbl)
                            n261 = xnode "Motors"() -> ("Motor"=w1065:T1)
                            n262 = local write "Large/Steel 3"(w1074) -> ()
                            n263 = xnode "Move a Fixed Distance"("Speed 1"=i8 20, "Distance 1"=w1064, "Motors"=w1065) -> ("NXT/EV3"=w1059:T3)  [unwired: 1 in]
                            n264 = xnode "Motors"() -> ("Motor"=w1067:T1)
                            n265 = xnode "Move a Fixed Distance"("Speed 1"=i8 -30, "Distance 1"=180, "Motors"=w1067, "NXT/EV3"=w1059) -> ("NXT/EV3"=w1058:T3)
                            n266 = call-poly <vilib>:"PolyWait.vi"("Time (1 sec)"=sgl 2.0, "NXT/EV3"=w1058) -> ("NXT/EV3"=w1060:T3)  [unwired: 2 in]
                            n267 = xnode "Motors"() -> ("Motor"=w1062:T1)
                            n268 = xnode "Move a Fixed Distance"("Speed 1"=i8 -20, "Distance 1"=w1064, "Motors"=w1062, "NXT/EV3"=w1060) -> ("NXT/EV3"=w1063:T3)
                            n269 = xnode "Motors"() -> ("Motor"=w1070:T1)
                            n270 = xnode "Move a Fixed Distance"("Speed 1"=i8 30, "Distance 1"=180, "Motors"=w1070, "NXT/EV3"=w1063) -> ()  [unwired: 1 out]
                          }
                        }
                      }
                      frame "Steel/HDPE" {
                        n271 = local read "Large/Steel 3"() -> (w1121:dbl)
                        n272 = Greater?(x=w1121, y=0.0) -> (0:w1122:bool)
                        n273 = case shown="False" w1122 {
                          frame False {
                            n274 = local read "Small/HDPE 3"() -> (w1124:dbl)
                            n275 = Greater?(x=w1124, y=0.0) -> (0:w1125:bool)
                            n276 = case shown="True" w1125 {
                              frame False {
                                (unwired) "labview wouldnt let me copy the variables successfully\nso I had to write every single case structure by hand."
                              }
                              frame True {
                                w1132 = 270 ("Distance 1")
                                n277 = local read "Small/HDPE 3"() -> (w1143:dbl)
                                n278 = xnode "Motors"() -> ("Motor"=w1133:T1)
                                n279 = xnode "Move a Fixed Distance"("Speed 1"=i8 20, "Distance 1"=w1132, "Motors"=w1133) -> ("NXT/EV3"=w1127:T3)  [unwired: 1 in]
                                n280 = Decrement(x=w1143) -> (x-1=w1142:dbl)
                                n281 = local write "Small/HDPE 3"(w1142) -> ()
                                n282 = xnode "Motors"() -> ("Motor"=w1135:T1)
                                n283 = xnode "Move a Fixed Distance"("Speed 1"=i8 -30, "Distance 1"=180, "Motors"=w1135, "NXT/EV3"=w1127) -> ("NXT/EV3"=w1126:T3)
                                n284 = call-poly <vilib>:"PolyWait.vi"("Time (1 sec)"=sgl 2.0, "NXT/EV3"=w1126) -> ("NXT/EV3"=w1128:T3)  [unwired: 2 in]
                                n285 = xnode "Motors"() -> ("Motor"=w1130:T1)
                                n286 = xnode "Move a Fixed Distance"("Speed 1"=i8 -20, "Distance 1"=w1132, "Motors"=w1130, "NXT/EV3"=w1128) -> ("NXT/EV3"=w1131:T3)
                                n287 = xnode "Motors"() -> ("Motor"=w1138:T1)
                                n288 = xnode "Move a Fixed Distance"("Speed 1"=i8 30, "Distance 1"=180, "Motors"=w1138, "NXT/EV3"=w1131) -> ()  [unwired: 1 out]
                              }
                            }
                          }
                          frame True {
                            w1194 = 150 ("Distance 1")
                            n289 = local read "Large/Steel 3"() -> (w1205:dbl)
                            n290 = xnode "Motors"() -> ("Motor"=w1195:T1)
                            n291 = xnode "Move a Fixed Distance"("Speed 1"=i8 20, "Distance 1"=w1194, "Motors"=w1195) -> ("NXT/EV3"=w1189:T3)  [unwired: 1 in]
                            n292 = xnode "Motors"() -> ("Motor"=w1197:T1)
                            n293 = xnode "Move a Fixed Distance"("Speed 1"=i8 -30, "Distance 1"=180, "Motors"=w1197, "NXT/EV3"=w1189) -> ("NXT/EV3"=w1188:T3)
                            n294 = Decrement(x=w1205) -> (x-1=w1204:dbl)
                            n295 = local write "Large/Steel 3"(w1204) -> ()
                            n296 = call-poly <vilib>:"PolyWait.vi"("Time (1 sec)"=sgl 2.0, "NXT/EV3"=w1188) -> ("NXT/EV3"=w1190:T3)  [unwired: 2 in]
                            n297 = xnode "Motors"() -> ("Motor"=w1192:T1)
                            n298 = xnode "Move a Fixed Distance"("Speed 1"=i8 -20, "Distance 1"=w1194, "Motors"=w1192, "NXT/EV3"=w1190) -> ("NXT/EV3"=w1193:T3)
                            n299 = xnode "Motors"() -> ("Motor"=w1200:T1)
                            n300 = xnode "Move a Fixed Distance"("Speed 1"=i8 30, "Distance 1"=180, "Motors"=w1200, "NXT/EV3"=w1193) -> ()  [unwired: 1 out]
                          }
                        }
                      }
                    }
                  }
                }
              }
              frame True {
                n301 = local read "Material 2"() -> (w1250:string)
                n302 = case shown="\"Steel/HDPE\"" w1250 {
                  frame "White Glass", Default {
                    n303 = local read "Large/Steel 2"() -> (w1253:dbl)
                    n304 = Greater?(x=w1253, y=0.0) -> (0:w1251:bool)
                    n305 = case shown="False" w1251 {
                      frame False {
                        n306 = local read "Small/HDPE 2"() -> (w1256:dbl)
                        n307 = Greater?(x=w1256, y=0.0) -> (0:w1254:bool)
                        n308 = case shown="True" w1254 {
                          frame False {
                            (unwired) "howdy random TA"
                          }
                          frame True {
                            w1263 = 220 ("Distance 1")
                            n309 = xnode "Motors"() -> ("Motor"=w1264:T1)
                            n310 = xnode "Move a Fixed Distance"("Speed 1"=i8 20, "Distance 1"=w1263, "Motors"=w1264) -> ("NXT/EV3"=w1258:T3)  [unwired: 1 in]
                            n311 = local read "Small/HDPE 2"() -> (w1274:dbl)
                            n312 = Decrement(x=w1274) -> (x-1=w1273:dbl)
                            n313 = local write "Small/HDPE 2"(w1273) -> ()
                            n314 = xnode "Motors"() -> ("Motor"=w1266:T1)
                            n315 = xnode "Move a Fixed Distance"("Speed 1"=i8 -30, "Distance 1"=180, "Motors"=w1266, "NXT/EV3"=w1258) -> ("NXT/EV3"=w1257:T3)
                            n316 = call-poly <vilib>:"PolyWait.vi"("Time (1 sec)"=sgl 2.0, "NXT/EV3"=w1257) -> ("NXT/EV3"=w1259:T3)  [unwired: 2 in]
                            n317 = xnode "Motors"() -> ("Motor"=w1261:T1)
                            n318 = xnode "Move a Fixed Distance"("Speed 1"=i8 -20, "Distance 1"=w1263, "Motors"=w1261, "NXT/EV3"=w1259) -> ("NXT/EV3"=w1262:T3)
                            n319 = xnode "Motors"() -> ("Motor"=w1269:T1)
                            n320 = xnode "Move a Fixed Distance"("Speed 1"=i8 30, "Distance 1"=180, "Motors"=w1269, "NXT/EV3"=w1262) -> ()  [unwired: 1 out]
                          }
                        }
                      }
                      frame True {
                        w1325 = 85 ("Distance 1")
                        n321 = local read "Large/Steel 2"() -> (w1336:dbl)
                        n322 = Decrement(x=w1336) -> (x-1=w1335:dbl)
                        n323 = xnode "Motors"() -> ("Motor"=w1326:T1)
                        n324 = local write "Large/Steel 2"(w1335) -> ()
                        n325 = xnode "Move a Fixed Distance"("Speed 1"=i8 20, "Distance 1"=w1325, "Motors"=w1326) -> ("NXT/EV3"=w1320:T3)  [unwired: 1 in]
                        n326 = xnode "Motors"() -> ("Motor"=w1328:T1)
                        n327 = xnode "Move a Fixed Distance"("Speed 1"=i8 -30, "Distance 1"=180, "Motors"=w1328, "NXT/EV3"=w1320) -> ("NXT/EV3"=w1319:T3)
                        n328 = call-poly <vilib>:"PolyWait.vi"("Time (1 sec)"=sgl 2.0, "NXT/EV3"=w1319) -> ("NXT/EV3"=w1321:T3)  [unwired: 2 in]
                        n329 = xnode "Motors"() -> ("Motor"=w1323:T1)
                        n330 = xnode "Move a Fixed Distance"("Speed 1"=i8 -20, "Distance 1"=w1325, "Motors"=w1323, "NXT/EV3"=w1321) -> ("NXT/EV3"=w1324:T3)
                        n331 = xnode "Motors"() -> ("Motor"=w1331:T1)
                        n332 = xnode "Move a Fixed Distance"("Speed 1"=i8 30, "Distance 1"=180, "Motors"=w1331, "NXT/EV3"=w1324) -> ()  [unwired: 1 out]
                      }
                    }
                  }
                  frame "Blue Glass" {
                    n333 = local read "Large/Steel 2"() -> (w1383:dbl)
                    n334 = Greater?(x=w1383, y=0.0) -> (0:w1382:bool)
                    n335 = case shown="True" w1382 {
                      frame True {
                        w1390 = 330 ("Distance 1")
                        n336 = local read "Large/Steel 2"() -> (w1401:dbl)
                        n337 = Decrement(x=w1401) -> (x-1=w1400:dbl)
                        n338 = local write "Large/Steel 2"(w1400) -> ()
                        n339 = xnode "Motors"() -> ("Motor"=w1391:T1)
                        n340 = xnode "Move a Fixed Distance"("Speed 1"=i8 20, "Distance 1"=w1390, "Motors"=w1391) -> ("NXT/EV3"=w1385:T3)  [unwired: 1 in]
                        n341 = xnode "Motors"() -> ("Motor"=w1393:T1)
                        n342 = xnode "Move a Fixed Distance"("Speed 1"=i8 -30, "Distance 1"=180, "Motors"=w1393, "NXT/EV3"=w1385) -> ("NXT/EV3"=w1384:T3)
                        n343 = call-poly <vilib>:"PolyWait.vi"("Time (1 sec)"=sgl 2.0, "NXT/EV3"=w1384) -> ("NXT/EV3"=w1386:T3)  [unwired: 2 in]
                        n344 = xnode "Motors"() -> ("Motor"=w1388:T1)
                        n345 = xnode "Move a Fixed Distance"("Speed 1"=i8 -20, "Distance 1"=w1390, "Motors"=w1388, "NXT/EV3"=w1386) -> ("NXT/EV3"=w1389:T3)
                        n346 = xnode "Motors"() -> ("Motor"=w1396:T1)
                        n347 = xnode "Move a Fixed Distance"("Speed 1"=i8 30, "Distance 1"=180, "Motors"=w1396, "NXT/EV3"=w1389) -> ()  [unwired: 1 out]
                      }
                      frame False {
                        n348 = local read "Small/HDPE 2"() -> (w1448:dbl)
                        n349 = Greater?(x=w1448, y=0.0) -> (0:w1446:bool)
                        n350 = case shown="True" w1446 {
                          frame False {
                            (unwired) "This statement is false"
                          }
                          frame True {
                            w1455 = 390 ("Distance 1")
                            n351 = local read "Small/HDPE 2"() -> (w1466:dbl)
                            n352 = Decrement(x=w1466) -> (x-1=w1465:dbl)
                            n353 = xnode "Motors"() -> ("Motor"=w1456:T1)
                            n354 = xnode "Move a Fixed Distance"("Speed 1"=i8 20, "Distance 1"=w1455, "Motors"=w1456) -> ("NXT/EV3"=w1450:T3)  [unwired: 1 in]
                            n355 = local write "Small/HDPE 2"(w1465) -> ()
                            n356 = xnode "Motors"() -> ("Motor"=w1458:T1)
                            n357 = xnode "Move a Fixed Distance"("Speed 1"=i8 -30, "Distance 1"=180, "Motors"=w1458, "NXT/EV3"=w1450) -> ("NXT/EV3"=w1449:T3)
                            n358 = call-poly <vilib>:"PolyWait.vi"("Time (1 sec)"=sgl 2.0, "NXT/EV3"=w1449) -> ("NXT/EV3"=w1451:T3)  [unwired: 2 in]
                            n359 = xnode "Motors"() -> ("Motor"=w1453:T1)
                            n360 = xnode "Move a Fixed Distance"("Speed 1"=i8 -20, "Distance 1"=w1455, "Motors"=w1453, "NXT/EV3"=w1451) -> ("NXT/EV3"=w1454:T3)
                            n361 = xnode "Motors"() -> ("Motor"=w1461:T1)
                            n362 = xnode "Move a Fixed Distance"("Speed 1"=i8 30, "Distance 1"=180, "Motors"=w1461, "NXT/EV3"=w1454) -> ()  [unwired: 1 out]
                          }
                        }
                      }
                    }
                  }
                  frame "Red Glass" {
                    n363 = local read "Large/Steel 2"() -> (w1513:dbl)
                    n364 = Greater?(x=w1513, y=0.0) -> (0:w1511:bool)
                    n365 = case shown="True" w1511 {
                      frame False {
                        n366 = local read "Small/HDPE 2"() -> (w1516:dbl)
                        n367 = Greater?(x=w1516, y=0.0) -> (0:w1514:bool)
                        n368 = case shown="True" w1514 {
                          frame False {
                            (unwired) "I hate everything\n"
                          }
                          frame True {
                            w1523 = 520 ("Distance 1")
                            n369 = local read "Small/HDPE 2"() -> (w1534:dbl)
                            n370 = xnode "Motors"() -> ("Motor"=w1524:T1)
                            n371 = xnode "Move a Fixed Distance"("Speed 1"=i8 20, "Distance 1"=w1523, "Motors"=w1524) -> ("NXT/EV3"=w1518:T3)  [unwired: 1 in]
                            n372 = Decrement(x=w1534) -> (x-1=w1533:dbl)
                            n373 = local write "Small/HDPE 2"(w1533) -> ()
                            n374 = xnode "Motors"() -> ("Motor"=w1526:T1)
                            n375 = xnode "Move a Fixed Distance"("Speed 1"=i8 -30, "Distance 1"=180, "Motors"=w1526, "NXT/EV3"=w1518) -> ("NXT/EV3"=w1517:T3)
                            n376 = call-poly <vilib>:"PolyWait.vi"("Time (1 sec)"=sgl 2.0, "NXT/EV3"=w1517) -> ("NXT/EV3"=w1519:T3)  [unwired: 2 in]
                            n377 = xnode "Motors"() -> ("Motor"=w1521:T1)
                            n378 = xnode "Move a Fixed Distance"("Speed 1"=i8 -20, "Distance 1"=w1523, "Motors"=w1521, "NXT/EV3"=w1519) -> ("NXT/EV3"=w1522:T3)
                            n379 = xnode "Motors"() -> ("Motor"=w1529:T1)
                            n380 = xnode "Move a Fixed Distance"("Speed 1"=i8 30, "Distance 1"=180, "Motors"=w1529, "NXT/EV3"=w1522) -> ()  [unwired: 1 out]
                          }
                        }
                      }
                      frame True {
                        w1585 = 450 ("Distance 1")
                        n381 = xnode "Motors"() -> ("Motor"=w1586:T1)
                        n382 = local read "Large/Steel 2"() -> (w1596:dbl)
                        n383 = xnode "Move a Fixed Distance"("Speed 1"=i8 20, "Distance 1"=w1585, "Motors"=w1586) -> ("NXT/EV3"=w1580:T3)  [unwired: 1 in]
                        n384 = Decrement(x=w1596) -> (x-1=w1595:dbl)
                        n385 = local write "Large/Steel 2"(w1595) -> ()
                        n386 = xnode "Motors"() -> ("Motor"=w1588:T1)
                        n387 = xnode "Move a Fixed Distance"("Speed 1"=i8 -30, "Distance 1"=180, "Motors"=w1588, "NXT/EV3"=w1580) -> ("NXT/EV3"=w1579:T3)
                        n388 = call-poly <vilib>:"PolyWait.vi"("Time (1 sec)"=sgl 2.0, "NXT/EV3"=w1579) -> ("NXT/EV3"=w1581:T3)  [unwired: 2 in]
                        n389 = xnode "Motors"() -> ("Motor"=w1583:T1)
                        n390 = xnode "Move a Fixed Distance"("Speed 1"=i8 -20, "Distance 1"=w1585, "Motors"=w1583, "NXT/EV3"=w1581) -> ("NXT/EV3"=w1584:T3)
                        n391 = xnode "Motors"() -> ("Motor"=w1591:T1)
                        n392 = xnode "Move a Fixed Distance"("Speed 1"=i8 30, "Distance 1"=180, "Motors"=w1591, "NXT/EV3"=w1584) -> ()  [unwired: 1 out]
                      }
                    }
                  }
                  frame "Steel/HDPE" {
                    n393 = local read "Large/Steel 2"() -> (w1643:dbl)
                    n394 = Greater?(x=w1643, y=0.0) -> (0:w1641:bool)
                    n395 = case shown="True" w1641 {
                      frame False {
                        n396 = local read "Small/HDPE 2"() -> (w1646:dbl)
                        n397 = Greater?(x=w1646, y=0.0) -> (0:w1644:bool)
                        n398 = case shown="True" w1644 {
                          frame False {
                            (unwired) "I've lost all my marbles"
                          }
                          frame True {
                            w1653 = 270 ("Distance 1")
                            n399 = xnode "Motors"() -> ("Motor"=w1654:T1)
                            n400 = local read "Small/HDPE 2"() -> (w1664:dbl)
                            n401 = xnode "Move a Fixed Distance"("Speed 1"=i8 20, "Distance 1"=w1653, "Motors"=w1654) -> ("NXT/EV3"=w1648:T3)  [unwired: 1 in]
                            n402 = Decrement(x=w1664) -> (x-1=w1663:dbl)
                            n403 = local write "Small/HDPE 2"(w1663) -> ()
                            n404 = xnode "Motors"() -> ("Motor"=w1656:T1)
                            n405 = xnode "Move a Fixed Distance"("Speed 1"=i8 -30, "Distance 1"=180, "Motors"=w1656, "NXT/EV3"=w1648) -> ("NXT/EV3"=w1647:T3)
                            n406 = call-poly <vilib>:"PolyWait.vi"("Time (1 sec)"=sgl 2.0, "NXT/EV3"=w1647) -> ("NXT/EV3"=w1649:T3)  [unwired: 2 in]
                            n407 = xnode "Motors"() -> ("Motor"=w1651:T1)
                            n408 = xnode "Move a Fixed Distance"("Speed 1"=i8 -20, "Distance 1"=w1653, "Motors"=w1651, "NXT/EV3"=w1649) -> ("NXT/EV3"=w1652:T3)
                            n409 = xnode "Motors"() -> ("Motor"=w1659:T1)
                            n410 = xnode "Move a Fixed Distance"("Speed 1"=i8 30, "Distance 1"=180, "Motors"=w1659, "NXT/EV3"=w1652) -> ()  [unwired: 1 out]
                          }
                        }
                      }
                      frame True {
                        w1715 = 150 ("Distance 1")
                        n411 = local read "Large/Steel 2"() -> (w1726:dbl)
                        n412 = xnode "Motors"() -> ("Motor"=w1716:T1)
                        n413 = xnode "Move a Fixed Distance"("Speed 1"=i8 20, "Distance 1"=w1715, "Motors"=w1716) -> ("NXT/EV3"=w1710:T3)  [unwired: 1 in]
                        n414 = Decrement(x=w1726) -> (x-1=w1725:dbl)
                        n415 = local write "Large/Steel 2"(w1725) -> ()
                        n416 = xnode "Motors"() -> ("Motor"=w1718:T1)
                        n417 = xnode "Move a Fixed Distance"("Speed 1"=i8 -30, "Distance 1"=180, "Motors"=w1718, "NXT/EV3"=w1710) -> ("NXT/EV3"=w1709:T3)
                        n418 = call-poly <vilib>:"PolyWait.vi"("Time (1 sec)"=sgl 2.0, "NXT/EV3"=w1709) -> ("NXT/EV3"=w1711:T3)  [unwired: 2 in]
                        n419 = xnode "Motors"() -> ("Motor"=w1713:T1)
                        n420 = xnode "Move a Fixed Distance"("Speed 1"=i8 -20, "Distance 1"=w1715, "Motors"=w1713, "NXT/EV3"=w1711) -> ("NXT/EV3"=w1714:T3)
                        n421 = xnode "Motors"() -> ("Motor"=w1721:T1)
                        n422 = xnode "Move a Fixed Distance"("Speed 1"=i8 30, "Distance 1"=180, "Motors"=w1721, "NXT/EV3"=w1714) -> ()  [unwired: 1 out]
                      }
                    }
                  }
                }
              }
            }
          }
          frame True {
            n423 = local read "Material 1"() -> (w1771:string)
            n424 = case shown="\"Steel/HDPE\"" w1771 {
              frame "White Glass", Default {
                n425 = local read "Large/Steel 1"() -> (w1773:dbl)
                n426 = Greater?(x=w1773, y=0.0) -> (0:w1772:bool)
                n427 = case shown="False" w1772 {
                  frame False {
                    n428 = local read "Small/HDPE 1"() -> (w1776:dbl)
                    n429 = Greater?(x=w1776, y=0.0) -> (0:w1775:bool)
                    n430 = case shown="True" w1775 {
                      frame False {
                        (unwired) "go away"
                      }
                      frame True {
                        w1784 = 220 ("Distance 1")
                        n431 = xnode "Motors"() -> ("Motor"=w1785:T1)
                        n432 = xnode "Move a Fixed Distance"("Speed 1"=i8 20, "Distance 1"=w1784, "Motors"=w1785) -> ("NXT/EV3"=w1779:T3)  [unwired: 1 in]
                        n433 = local read "Small/HDPE 1"() -> (w1795:dbl)
                        n434 = Decrement(x=w1795) -> (x-1=w1794:dbl)
                        n435 = local write "Small/HDPE 1"(w1794) -> ()
                        n436 = xnode "Motors"() -> ("Motor"=w1787:T1)
                        n437 = xnode "Move a Fixed Distance"("Speed 1"=i8 -30, "Distance 1"=180, "Motors"=w1787, "NXT/EV3"=w1779) -> ("NXT/EV3"=w1778:T3)
                        n438 = call-poly <vilib>:"PolyWait.vi"("Time (1 sec)"=sgl 2.0, "NXT/EV3"=w1778) -> ("NXT/EV3"=w1780:T3)  [unwired: 2 in]
                        n439 = xnode "Motors"() -> ("Motor"=w1782:T1)
                        n440 = xnode "Move a Fixed Distance"("Speed 1"=i8 -20, "Distance 1"=w1784, "Motors"=w1782, "NXT/EV3"=w1780) -> ("NXT/EV3"=w1783:T3)
                        n441 = xnode "Motors"() -> ("Motor"=w1790:T1)
                        n442 = xnode "Move a Fixed Distance"("Speed 1"=i8 30, "Distance 1"=180, "Motors"=w1790, "NXT/EV3"=w1783) -> ()  [unwired: 1 out]
                      }
                    }
                  }
                  frame True {
                    w1846 = 85 ("Distance 1")
                    n443 = local read "Large/Steel 1"() -> (w1857:dbl)
                    n444 = Decrement(x=w1857) -> (x-1=w1856:dbl)
                    n445 = local write "Large/Steel 1"(w1856) -> ()
                    n446 = xnode "Motors"() -> ("Motor"=w1847:T1)
                    n447 = xnode "Move a Fixed Distance"("Speed 1"=i8 20, "Distance 1"=w1846, "Motors"=w1847) -> ("NXT/EV3"=w1841:T3)  [unwired: 1 in]
                    n448 = xnode "Motors"() -> ("Motor"=w1849:T1)
                    n449 = xnode "Move a Fixed Distance"("Speed 1"=i8 -30, "Distance 1"=180, "Motors"=w1849, "NXT/EV3"=w1841) -> ("NXT/EV3"=w1840:T3)
                    n450 = call-poly <vilib>:"PolyWait.vi"("Time (1 sec)"=sgl 2.0, "NXT/EV3"=w1840) -> ("NXT/EV3"=w1842:T3)  [unwired: 2 in]
                    n451 = xnode "Motors"() -> ("Motor"=w1844:T1)
                    n452 = xnode "Move a Fixed Distance"("Speed 1"=i8 -20, "Distance 1"=w1846, "Motors"=w1844, "NXT/EV3"=w1842) -> ("NXT/EV3"=w1845:T3)
                    n453 = xnode "Motors"() -> ("Motor"=w1852:T1)
                    n454 = xnode "Move a Fixed Distance"("Speed 1"=i8 30, "Distance 1"=180, "Motors"=w1852, "NXT/EV3"=w1845) -> ()  [unwired: 1 out]
                  }
                }
              }
              frame "Red Glass" {
                n455 = local read "Large/Steel 1"() -> (w1904:dbl)
                n456 = Greater?(x=w1904, y=0.0) -> (0:w1903:bool)
                n457 = case shown="True" w1903 {
                  frame False {
                    n458 = local read "Small/HDPE 1"() -> (w1907:dbl)
                    n459 = Greater?(x=w1907, y=0.0) -> (0:w1905:bool)
                    n460 = case shown="True" w1905 {
                      frame False {
                        (unwired) "donezo"
                      }
                      frame True {
                        w1914 = 520 ("Distance 1")
                        n461 = local read "Small/HDPE 1"() -> (w1925:dbl)
                        n462 = xnode "Motors"() -> ("Motor"=w1915:T1)
                        n463 = Decrement(x=w1925) -> (x-1=w1924:dbl)
                        n464 = xnode "Move a Fixed Distance"("Speed 1"=i8 20, "Distance 1"=w1914, "Motors"=w1915) -> ("NXT/EV3"=w1909:T3)  [unwired: 1 in]
                        n465 = local write "Small/HDPE 1"(w1924) -> ()
                        n466 = xnode "Motors"() -> ("Motor"=w1917:T1)
                        n467 = xnode "Move a Fixed Distance"("Speed 1"=i8 -30, "Distance 1"=180, "Motors"=w1917, "NXT/EV3"=w1909) -> ("NXT/EV3"=w1908:T3)
                        n468 = call-poly <vilib>:"PolyWait.vi"("Time (1 sec)"=sgl 2.0, "NXT/EV3"=w1908) -> ("NXT/EV3"=w1910:T3)  [unwired: 2 in]
                        n469 = xnode "Motors"() -> ("Motor"=w1912:T1)
                        n470 = xnode "Move a Fixed Distance"("Speed 1"=i8 -20, "Distance 1"=w1914, "Motors"=w1912, "NXT/EV3"=w1910) -> ("NXT/EV3"=w1913:T3)
                        n471 = xnode "Motors"() -> ("Motor"=w1920:T1)
                        n472 = xnode "Move a Fixed Distance"("Speed 1"=i8 30, "Distance 1"=180, "Motors"=w1920, "NXT/EV3"=w1913) -> ()  [unwired: 1 out]
                      }
                    }
                  }
                  frame True {
                    w1976 = 450 ("Distance 1")
                    n473 = local read "Large/Steel 1"() -> (w1987:dbl)
                    n474 = xnode "Motors"() -> ("Motor"=w1977:T1)
                    n475 = Decrement(x=w1987) -> (x-1=w1986:dbl)
                    n476 = xnode "Move a Fixed Distance"("Speed 1"=i8 20, "Distance 1"=w1976, "Motors"=w1977) -> ("NXT/EV3"=w1971:T3)  [unwired: 1 in]
                    n477 = local write "Large/Steel 1"(w1986) -> ()
                    n478 = xnode "Motors"() -> ("Motor"=w1979:T1)
                    n479 = xnode "Move a Fixed Distance"("Speed 1"=i8 -30, "Distance 1"=180, "Motors"=w1979, "NXT/EV3"=w1971) -> ("NXT/EV3"=w1970:T3)
                    n480 = call-poly <vilib>:"PolyWait.vi"("Time (1 sec)"=sgl 2.0, "NXT/EV3"=w1970) -> ("NXT/EV3"=w1972:T3)  [unwired: 2 in]
                    n481 = xnode "Motors"() -> ("Motor"=w1974:T1)
                    n482 = xnode "Move a Fixed Distance"("Speed 1"=i8 -20, "Distance 1"=w1976, "Motors"=w1974, "NXT/EV3"=w1972) -> ("NXT/EV3"=w1975:T3)
                    n483 = xnode "Motors"() -> ("Motor"=w1982:T1)
                    n484 = xnode "Move a Fixed Distance"("Speed 1"=i8 30, "Distance 1"=180, "Motors"=w1982, "NXT/EV3"=w1975) -> ()  [unwired: 1 out]
                  }
                }
              }
              frame "Blue Glass" {
                n485 = local read "Large/Steel 1"() -> (w2034:dbl)
                n486 = Greater?(x=w2034, y=0.0) -> (0:w2032:bool)
                n487 = case shown="False" w2032 {
                  frame False {
                    n488 = local read "Small/HDPE 1"() -> (w2036:dbl)
                    n489 = Greater?(x=w2036, y=0.0) -> (0:w2037:bool)
                    n490 = case shown="True" w2037 {
                      frame False {
                        (unwired) "Welcome to labview hell"
                      }
                      frame True {
                        w2044 = 390 ("Distance 1")
                        n491 = local read "Small/HDPE 1"() -> (w2055:dbl)
                        n492 = xnode "Motors"() -> ("Motor"=w2045:T1)
                        n493 = xnode "Move a Fixed Distance"("Speed 1"=i8 20, "Distance 1"=w2044, "Motors"=w2045) -> ("NXT/EV3"=w2039:T3)  [unwired: 1 in]
                        n494 = Decrement(x=w2055) -> (x-1=w2054:dbl)
                        n495 = local write "Small/HDPE 1"(w2054) -> ()
                        n496 = xnode "Motors"() -> ("Motor"=w2047:T1)
                        n497 = xnode "Move a Fixed Distance"("Speed 1"=i8 -30, "Distance 1"=180, "Motors"=w2047, "NXT/EV3"=w2039) -> ("NXT/EV3"=w2038:T3)
                        n498 = call-poly <vilib>:"PolyWait.vi"("Time (1 sec)"=sgl 2.0, "NXT/EV3"=w2038) -> ("NXT/EV3"=w2040:T3)  [unwired: 2 in]
                        n499 = xnode "Motors"() -> ("Motor"=w2042:T1)
                        n500 = xnode "Move a Fixed Distance"("Speed 1"=i8 -20, "Distance 1"=w2044, "Motors"=w2042, "NXT/EV3"=w2040) -> ("NXT/EV3"=w2043:T3)
                        n501 = xnode "Motors"() -> ("Motor"=w2050:T1)
                        n502 = xnode "Move a Fixed Distance"("Speed 1"=i8 30, "Distance 1"=180, "Motors"=w2050, "NXT/EV3"=w2043) -> ()  [unwired: 1 out]
                      }
                    }
                  }
                  frame True {
                    w2106 = 330 ("Distance 1")
                    n503 = local read "Large/Steel 1"() -> (w2117:dbl)
                    n504 = xnode "Motors"() -> ("Motor"=w2107:T1)
                    n505 = xnode "Move a Fixed Distance"("Speed 1"=i8 20, "Distance 1"=w2106, "Motors"=w2107) -> ("NXT/EV3"=w2101:T3)  [unwired: 1 in]
                    n506 = Decrement(x=w2117) -> (x-1=w2116:dbl)
                    n507 = local write "Large/Steel 1"(w2116) -> ()
                    n508 = xnode "Motors"() -> ("Motor"=w2109:T1)
                    n509 = xnode "Move a Fixed Distance"("Speed 1"=i8 -30, "Distance 1"=180, "Motors"=w2109, "NXT/EV3"=w2101) -> ("NXT/EV3"=w2100:T3)
                    n510 = call-poly <vilib>:"PolyWait.vi"("Time (1 sec)"=sgl 2.0, "NXT/EV3"=w2100) -> ("NXT/EV3"=w2102:T3)  [unwired: 2 in]
                    n511 = xnode "Motors"() -> ("Motor"=w2104:T1)
                    n512 = xnode "Move a Fixed Distance"("Speed 1"=i8 -20, "Distance 1"=w2106, "Motors"=w2104, "NXT/EV3"=w2102) -> ("NXT/EV3"=w2105:T3)
                    n513 = xnode "Motors"() -> ("Motor"=w2112:T1)
                    n514 = xnode "Move a Fixed Distance"("Speed 1"=i8 30, "Distance 1"=180, "Motors"=w2112, "NXT/EV3"=w2105) -> ()  [unwired: 1 out]
                  }
                }
              }
              frame "Steel/HDPE" {
                n515 = local read "Large/Steel 1"() -> (w2164:dbl)
                n516 = Greater?(x=w2164, y=0.0) -> (0:w2163:bool)
                n517 = case shown="False" w2163 {
                  frame False {
                    n518 = local read "Small/HDPE 1"() -> (w2167:dbl)
                    n519 = Greater?(x=w2167, y=0.0) -> (0:w2166:bool)
                    n520 = case shown="True" w2166 {
                      frame False {
                        (unwired) "why are you even here"
                      }
                      frame True {
                        w2174 = 270 ("Distance 1")
                        n521 = local read "Small/HDPE 1"() -> (w2185:dbl)
                        n522 = xnode "Motors"() -> ("Motor"=w2175:T1)
                        n523 = xnode "Move a Fixed Distance"("Speed 1"=i8 20, "Distance 1"=w2174, "Motors"=w2175) -> ("NXT/EV3"=w2169:T3)  [unwired: 1 in]
                        n524 = Decrement(x=w2185) -> (x-1=w2184:dbl)
                        n525 = local write "Small/HDPE 1"(w2184) -> ()
                        n526 = xnode "Motors"() -> ("Motor"=w2177:T1)
                        n527 = xnode "Move a Fixed Distance"("Speed 1"=i8 -30, "Distance 1"=180, "Motors"=w2177, "NXT/EV3"=w2169) -> ("NXT/EV3"=w2168:T3)
                        n528 = call-poly <vilib>:"PolyWait.vi"("Time (1 sec)"=sgl 2.0, "NXT/EV3"=w2168) -> ("NXT/EV3"=w2170:T3)  [unwired: 2 in]
                        n529 = xnode "Motors"() -> ("Motor"=w2172:T1)
                        n530 = xnode "Move a Fixed Distance"("Speed 1"=i8 -20, "Distance 1"=w2174, "Motors"=w2172, "NXT/EV3"=w2170) -> ("NXT/EV3"=w2173:T3)
                        n531 = xnode "Motors"() -> ("Motor"=w2180:T1)
                        n532 = xnode "Move a Fixed Distance"("Speed 1"=i8 30, "Distance 1"=180, "Motors"=w2180, "NXT/EV3"=w2173) -> ()  [unwired: 1 out]
                      }
                    }
                  }
                  frame True {
                    w2236 = 150 ("Distance 1")
                    n533 = local read "Large/Steel 1"() -> (w2247:dbl)
                    n534 = xnode "Motors"() -> ("Motor"=w2237:T1)
                    n535 = xnode "Move a Fixed Distance"("Speed 1"=i8 20, "Distance 1"=w2236, "Motors"=w2237) -> ("NXT/EV3"=w2231:T3)  [unwired: 1 in]
                    n536 = Decrement(x=w2247) -> (x-1=w2246:dbl)
                    n537 = xnode "Motors"() -> ("Motor"=w2239:T1)
                    n538 = xnode "Move a Fixed Distance"("Speed 1"=i8 -30, "Distance 1"=180, "Motors"=w2239, "NXT/EV3"=w2231) -> ("NXT/EV3"=w2230:T3)
                    n539 = local write "Large/Steel 1"(w2246) -> ()
                    n540 = call-poly <vilib>:"PolyWait.vi"("Time (1 sec)"=sgl 2.0, "NXT/EV3"=w2230) -> ("NXT/EV3"=w2232:T3)  [unwired: 2 in]
                    n541 = xnode "Motors"() -> ("Motor"=w2234:T1)
                    n542 = xnode "Move a Fixed Distance"("Speed 1"=i8 -20, "Distance 1"=w2236, "Motors"=w2234, "NXT/EV3"=w2232) -> ("NXT/EV3"=w2235:T3)
                    n543 = xnode "Motors"() -> ("Motor"=w2242:T1)
                    n544 = xnode "Move a Fixed Distance"("Speed 1"=i8 30, "Distance 1"=180, "Motors"=w2242, "NXT/EV3"=w2235) -> ()  [unwired: 1 out]
                  }
                }
              }
            }
          }
        }
      }
    }
  }
